vi "Null Broadcast Events--constant.vi"() -> (3 "RaspberryPiPico Broadcast Events":T1)   [LabVIEW 2020, in "RaspberryPiPico.lvlib"]
doc: "Returns the broadcast events cluster with null references for defining the event types in a Register For Events function.\n_____\nBased on DQMH Dev Tools: Project Template 7.1.0.1503."
uses:
  RaspberryPiPico.lvlib
  Broadcast Events--cluster.ctl
  Did Init Argument--cluster.ctl
  Status Updated Argument--cluster.ctl
  Error Reported Argument--cluster.ctl
  Stop Argument--cluster.ctl
  Get Module Execution Status Argument--cluster.ctl
  Instrument Connected Argument--cluster.ctl
  Analog Inputs Updated Argument--cluster.ctl
  Digital Inputs Updated Argument--cluster.ctl
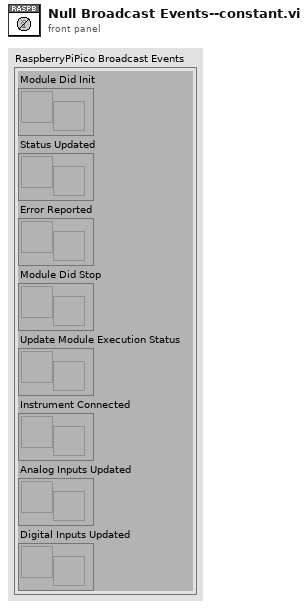
[diagram p1: front panel]
types:
  T1 = typedef "RaspberryPiPico.lvlib/Broadcast Events--cluster.ctl" = cluster{"Module Did Init":refnum<user-event>, "Status Updated":refnum<user-event>, "Error Reported":refnum<user-event>, "Module Did Stop":refnum<user-event>, "Update Module Execution Status":refnum<user-event>, "Instrument Connected":refnum<user-event>, "Analog Inputs Updated":refnum<user-event>, "Digital Inputs Updated":refnum<user-event>}
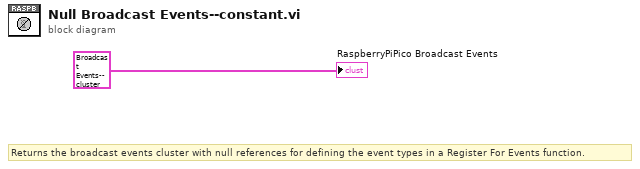
[diagram p0: block diagram]
diagram:
  # "Returns the broadcast events cluster with null references for defining the event types in a Register For Events function."
  "RaspberryPiPico Broadcast Events" <- T1 {"Module Did Init"=refnum, "Status Updated"=refnum, "Error Reported"=refnum, "Module Did Stop"=refnum, "Update Module Execution Status"=refnum, "Instrument Connected"=refnum, "Analog Inputs Updated"=refnum, "Digital Inputs Updated"=refnum} ("Broadcast Events")
